vi "number1-bubble sort.vi"(3 "Boolean":bool=TRUE, 4 "Array":dbl[](array[numeric]), 5 "wait":u32=10) -> (1 "Waveform Graph":dbl[](graph))   [LabVIEW 2014]
doc: "This VI implements bubble sort fully programmed in LabVIEW. In addition, it allows you to set a wait in the main loop and displays the partially sorted array so that you can see the actual process that bubble sort takes to sort the array"
panel:
  in  "Number of Elements":i32=1024
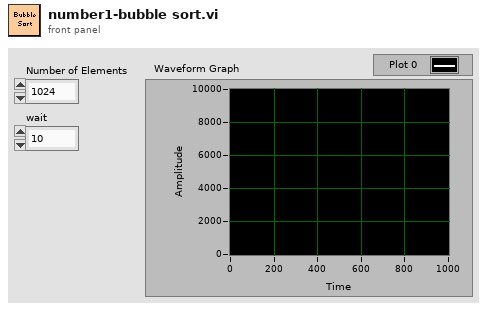
[diagram p1: front panel]
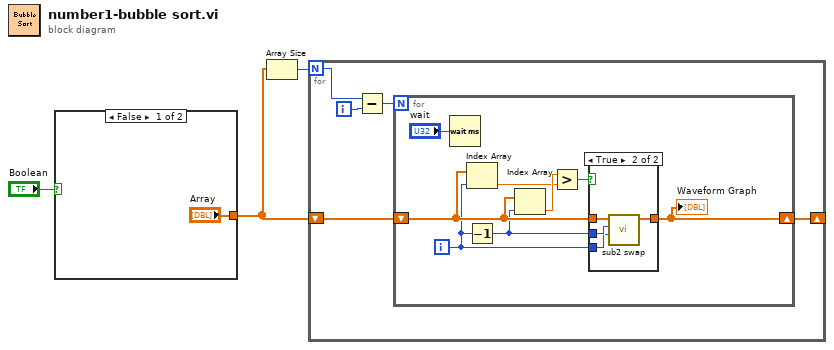
[diagram p0: block diagram]
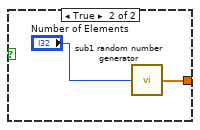
[diagram p2: hidden frame]
diagram:
  n1 = case shown="False" "Boolean" {
    tunnel: ["Array" w6] -> w2
    frame False {
    }
    frame True {
      n2 = call "sub1 random number generator.vi"("Numeric"="Number of Elements") -> ("Array"=w6:dbl[])  [unwired: 4 in]
    }
  }
  n3 = Array Size(array=w2) -> (size(s)=w3:i32)
  n4 = for {
    N: w3 -> [w10]
    shift-right: [w11] -> _
    shift-left: w2 -> [w7]
    i -> [w8]
    n5 = Subtract(x=w10, y=w8) -> (x-y=w9:i32)
    n6 = for {
      N: w9 -> [_]
      shift-right: [w13] -> w11
      shift-left: w7 -> [w18]
      i -> [w15]
      n7 = Wait (ms)(milliseconds to wait="wait") -> ()  [unwired: 1 out]
      n8 = Index Array(array=w18, index=w15) -> (element=w16:dbl)
      n9 = Decrement(x=w15) -> (x-1=w14:i32)
      n10 = Index Array(array=w18, index=w14) -> (element=w17:dbl)
      n11 = Greater?(x=w17, y=w16) -> (0:w19:bool)
      n12 = case shown="True" w19 {
        tunnel: w18 -> [w20 w24]
        tunnel: w14 -> [_ w23]
        tunnel: w15 -> [_ w22]
        tunnel: [w20 w21] -> w13
        frame False {
        }
        frame True {
          n13 = call "sub2 swap.vi"("Y"=w22, "X"=w23, "Original"=w24) -> ("After Swapped"=w21:dbl[])  [unwired: 4 in]
        }
      }
      "Waveform Graph" <- w13
    }
  }
